vi "reward_behavior_michelle_visjitter_conswin_AllEnticefx.vi"() -> ()   [LabVIEW 2019]
doc: "The myRIO Project template acquires acceleration data from the onboard accelerometer and displays the changes of acceleration values in a waveform chart."
uses:
  <vilib>/myRIO/Common/Instrument Driver Framework/Utilities/typedefs/Generic FPGA Reference.ctl
  <vilib>/myRIO/Common/Instrument Driver Framework/Utilities/typedefs/myRIO v1.0 Reference.ctl
  <vilib>/myRIO/Common/Instrument Driver Framework/Utilities/typedefs/Hardware Version Enum.ctl
  <vilib>/myRIO/Common/Instrument Driver Framework/Utilities/typedefs/myRIO Generic Hardware Reference.ctl
  <vilib>/userdefined/High Color/nirio_resource_hc.ctl
  <vilib>/myRIO/Common/Instrument Driver Framework/Utilities/vis/Is FPGA Ref Available.vi
  <vilib>/myRIO/Common/Instrument Driver Framework/myRIO v1.0/Encoder/typedefs/Encoder Signal Mode.ctl
  <vilib>/myRIO/Common/Instrument Driver Framework/myRIO v1.0/Encoder/typedefs/Encoder Channels Enum.ctl
  <vilib>/myRIO/Instrument Drivers/Onboard IO/Encoder/typedefs/Encoder Reference.ctl
  <vilib>/myRIO/Instrument Drivers/Onboard IO/Encoder/Encoder.lvlib
  <vilib>/myRIO/Instrument Drivers/Onboard IO/Encoder/vis/Read.vi
  <vilib>/myRIO/Common/Instrument Driver Framework/myRIO v1.0/Encoder/typedefs/Encoder Configuration v1.0.ctl
  <vilib>/myRIO/Common/Instrument Driver Framework/myRIO v1.0/Encoder/vis/myRIO v1.1 Open Encoder.vi
  <vilib>/myRIO/Common/Instrument Driver Framework/myRIO v1.0/Encoder/vis/myRIO v1.0 Configure Encoder.vi
  <vilib>/myRIO/Instrument Drivers/Onboard IO/Encoder/vis/myRIO Encoder Open.xnode
  <vilib>/myRIO/Express VI/Onboard IO/Encoder/Encoder Express VI.xnode
  <vilib>/myRIO/Express VI/Onboard IO/DI/DI Express VI.xnode
  <vilib>/myRIO/Instrument Drivers/Onboard IO/DIO/vis/Read.vi
  <vilib>/myRIO/Instrument Drivers/Onboard IO/DIO/DIO.lvlib
  <vilib>/myRIO/Common/Instrument Driver Framework/myRIO v1.0/DIO/typedefs/DIO Channels Enum.ctl
  <vilib>/myRIO/Common/Instrument Driver Framework/myRIO v1.0/DIO/typedefs/DIO Channels List.ctl
  <vilib>/myRIO/Instrument Drivers/Onboard IO/DIO/typedefs/DIO Reference.ctl
  <vilib>/myRIO/Instrument Drivers/Onboard IO/DIO/vis/myRIO DIO Open.xnode
  <vilib>/myRIO/Common/Instrument Driver Framework/myRIO v1.0/DIO/vis/myRIO v1.1 Open DIO.vi
  <vilib>/myRIO/Instrument Drivers/Onboard IO/DIO/vis/Write.vi
  <vilib>/myRIO/Express VI/Onboard IO/DO/DO Express VI.xnode
  <vilib>/Analysis/Matrix/Datatypes/RealMatrix.ctl
  <vilib>/Analysis/Matrix/NI_Matrix.lvlib
panel:
  out "ContrastChoice":dbl
  out "MissCrit":i32
  out "EnticeMatch":i32
  out "CatchVal":i32
  out "Enticements":i32
  in  "Entice":bool
  out "Misses":i32
  out "GoAhead":bool
  out "TimeOutDuration":i32
  out "ActiveTime":dbl
  out "ConsumptionGo":bool=TRUE
  out "Consumption_Period":i32
  out "Watch_Display":bool=TRUE
  in  "Give reward":bool
  out "Timings":dbl[](array[numeric])
  out "ISI":dbl
  out "ISI start time":dbl
  out "Time_out":bool=TRUE
  out "Time since lick":dbl
  out "Time of last lick":dbl
  out "Rewarded trials":dbl[](array[numeric])
  out "Rewards":u16
  out "Active Trial":bool
  out "Array temp2":T1
  out "Stimuli Loaded":bool
  out "Stim_ID":dbl[](array[numeric])
  out "Reward_mat":dbl[](array[numeric])
  out "Reward":bool=TRUE
  out "Frame clock":i32
  out "Licks":u32
  out "Lick":bool
  out "Time":dbl
  out "Stop":bool
  in  "Frames to collect":u32
  out "Overflow?":bool
  out "Counter Value":i32
  out "Velocity":dbl
  out "Velocity Plot":dbl[](graph)
  out "Velocity array":dbl[](array[numeric])
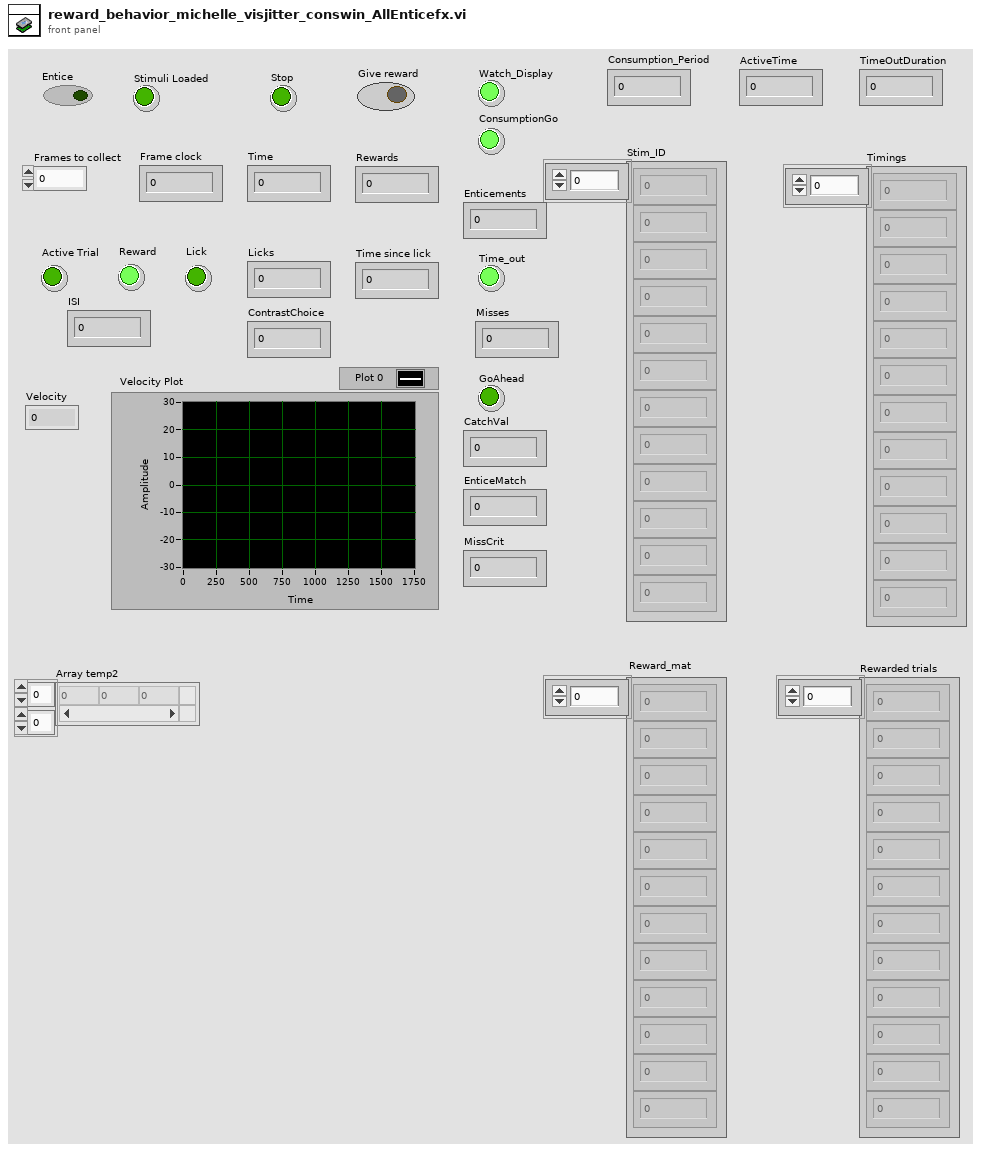
[diagram p1: front panel]
types:
  T1 = typedef "NI_Matrix.lvlib/RealMatrix.ctl" = dbl[][]
  T2 = typedef "Encoder.lvlib/Encoder Reference.ctl" = cluster{"myRIO Reference":T3, "Encoder Channels Enum":T7}
  T3 = typedef "myRIO Generic Hardware Reference.ctl" = cluster{"myRIO Model":T4, "myRIO Hardware Reference":T5}
  T4 = typedef "Hardware Version Enum.ctl" = enum16{"Unknown", "myRIO-1900", "myRIO-1950", "roboRIO", "NI ELVIS RIO CM", "ELVIS III"}
  T5 = typedef "myRIO v1.0 Reference.ctl" = cluster{"Generic FPGA Reference":T6, "Allow multiple opens":bool}
  T6 = typedef "Generic FPGA Reference.ctl" = refnum<k20>
  T7 = typedef "Encoder Channels Enum.ctl" = enum16{"Not Connected", "C/ENC0", "C/ENC1", "A/ENC", "A/ENC0", "A/ENC1", "A/ENC2", "A/ENC3", "A/ENC4", "A/ENC5", "A/ENC6", "A/ENC7", "A/ENC8", "A/ENC9", "B/ENC", "B/ENC0", "B/ENC1", "B/ENC2", "B/ENC3", "B/ENC4", "B/ENC5", "B/ENC6", "B/ENC7", "B/ENC8", "B/ENC9", "DIO/ENC0", "DIO/ENC1", "DIO/ENC2", "DIO/ENC3", "DIO/ENC4"}
  T8 = typedef "Encoder Signal Mode.ctl" = enum16{"Quadrature phase signal", "Step and direction signal"}
  T9 = typedef "nirio_resource_hc.ctl" = tag
  T10 = typedef "DIO.lvlib/DIO Reference.ctl" = cluster{"myRIO Reference":T3, "DIO Channels List":T11}
  T11 = typedef "DIO Channels List.ctl" = T12[]
  T12 = typedef "DIO Channels Enum.ctl" = enum16{"Not Connected", "C/DIO0", "C/DIO1", "C/DIO2", "C/DIO3", "C/DIO4", "C/DIO5", "C/DIO6", "C/DIO7", "A/DIO0", "A/DIO1", "A/DIO2", "A/DIO3", "A/DIO4", "A/DIO5", "A/DIO6", "A/DIO7", "A/DIO8", "A/DIO9", "A/DIO10", "A/DIO11", "A/DIO12", "A/DIO13", "A/DIO14", "A/DIO15", "A/DIO16", "A/DIO17", "A/DIO18", "A/DIO19", "B/DIO0", "B/DIO1", "B/DIO2", "B/DIO3", "B/DIO4", "B/DIO5", "B/DIO6", "B/DIO7", "B/DIO8", "B/DIO9", "B/DIO10", "B/DIO11", "B/DIO12", "B/DIO13", "B/DIO14", "B/DIO15", "B/DIO16", "B/DIO17", "B/DIO18", "B/DIO19", "LED0", "LED1", "LED2", "LED3", "Button0", "DIO/DIO0", "DIO/DIO1", "DIO/DIO2", "DIO/DIO3", "DIO/DIO4", "DIO/DIO5", "DIO/DIO6", "DIO/DIO7", "DIO/DIO8", "DIO/DIO9", "SPI/CS0", "SPI/CS1", "SPI/CS2", "SPI/CS3", "LED RADIO (Green)", "LED RADIO (Red)", "LED COMM (Green)", "LED COMM (Red)", "LED MODE (Green)", "LED MODE (Red)"}
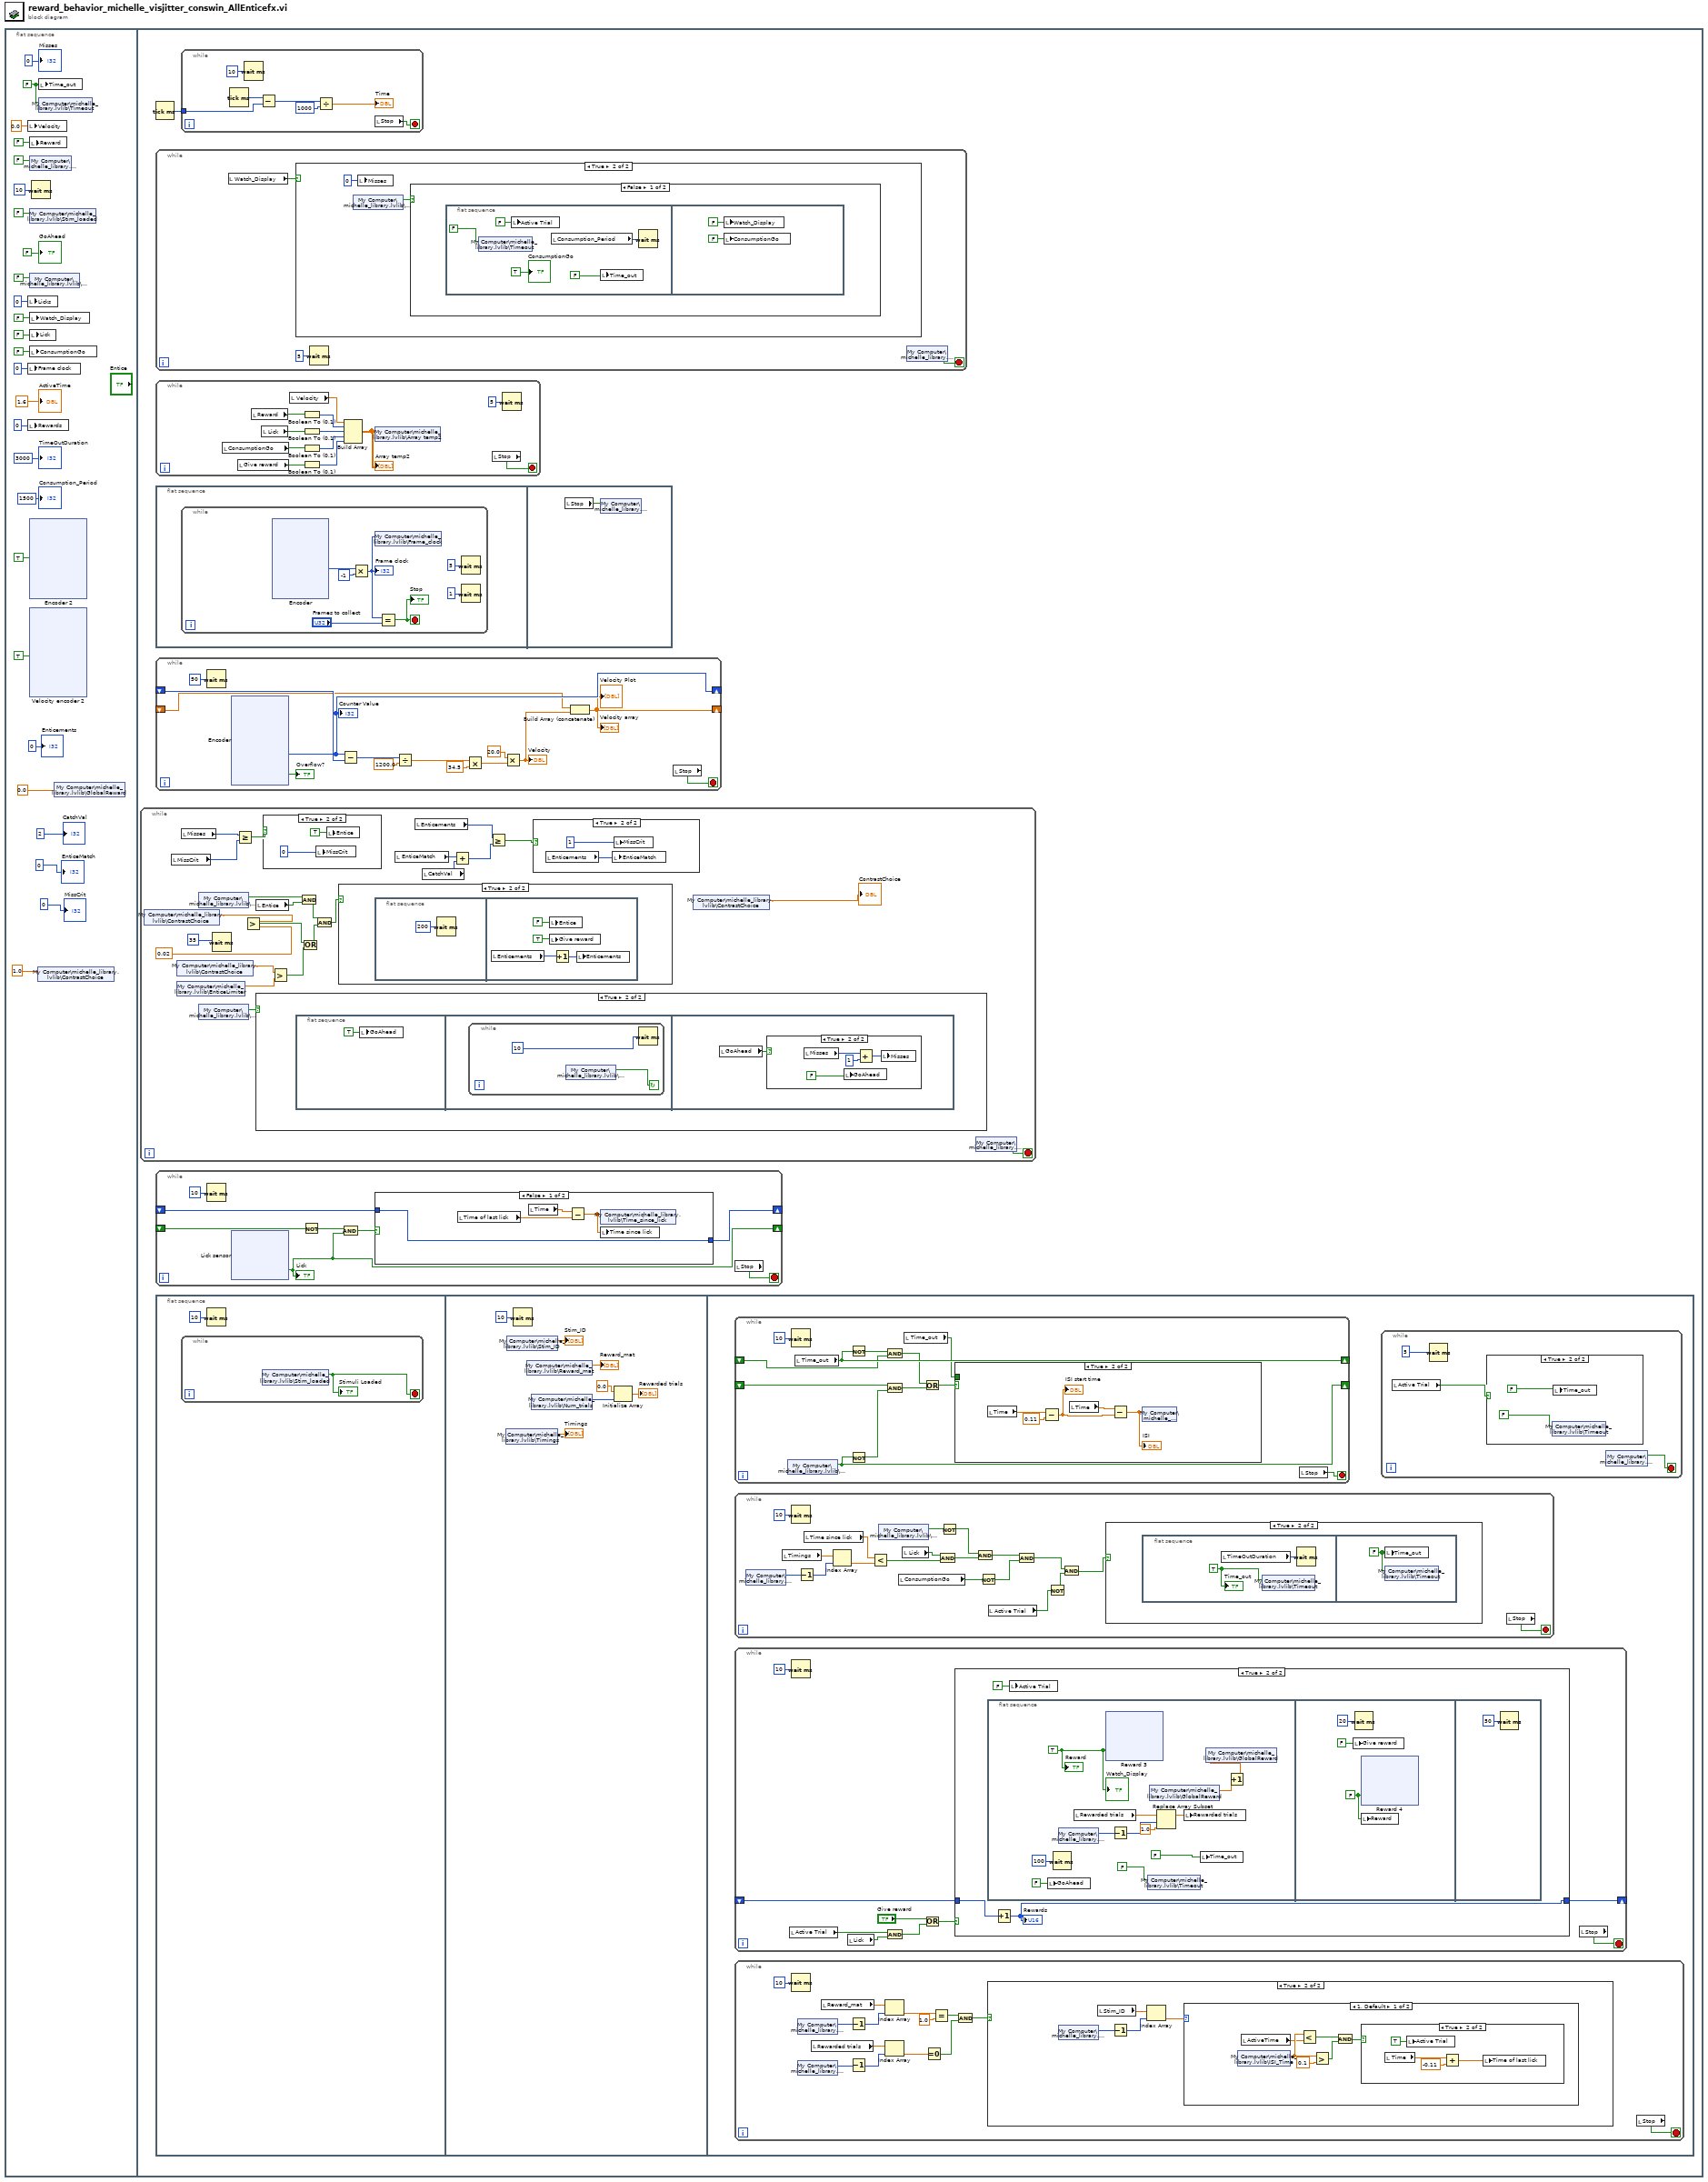
[diagram p0: block diagram]
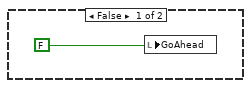
[diagram p5: hidden frame]
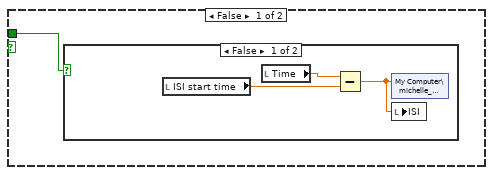
[diagram p11: hidden frame]
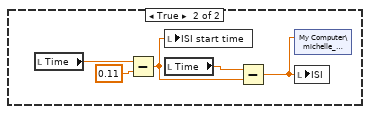
[diagram p12: hidden frame]
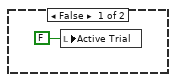
[diagram p13: hidden frame]
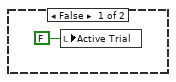
[diagram p14: hidden frame]
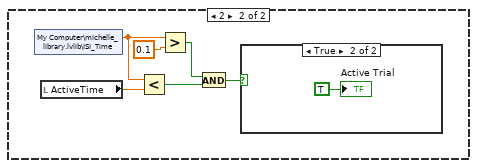
[diagram p15: hidden frame]
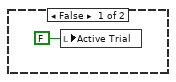
[diagram p16: hidden frame]
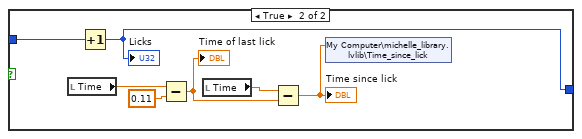
[diagram p18: hidden frame]
diagram:
  n1 = flat-sequence {
    frame #0 {
      w14 = FALSE ("Time_out")
      n2 = local write "Velocity"(0.0 ("Velocity")) -> ()
      n3 = local write "Licks"(u32 0 ("Licks")) -> ()
      n4 = local write "Frame clock"(u32 0 ("Frames")) -> ()
      n5 = local write "Rewards"(u16 0 ("Rewards")) -> ()
      n6 = local write "Reward"(FALSE ("Give reward")) -> ()
      n7 = shared-variable "My Computer\\michelle_library.lvlib\\Stop"(FALSE ("Stop")) -> ()  [unwired: 1 in, 1 out]
      n8 = shared-variable "My Computer\\michelle_library.lvlib\\Stim_loaded"(FALSE ("Stim_loaded")) -> ()  [unwired: 1 in, 1 out]
      n9 = shared-variable "My Computer\\michelle_library.lvlib\\Display"(FALSE ("Display")) -> ()  [unwired: 1 in, 1 out]
      n10 = local write "Watch_Display"(FALSE ("Watch_Display")) -> ()
      n11 = local write "Lick"(FALSE ("Lick")) -> ()
      n12 = local write "ConsumptionGo"(FALSE ("ConsumptionGo")) -> ()
      n13 = xnode "Encoder 2"("Reset Counter"=TRUE) -> ()  [unwired: 1 in, 4 out]
      n14 = xnode "Velocity encoder 2"("Reset Counter"=TRUE) -> ()  [unwired: 1 in, 4 out]
      n15 = Wait (ms)(milliseconds to wait=u32 10) -> ()  [unwired: 1 out]
      n16 = shared-variable "My Computer\\michelle_library.lvlib\\ContrastChoice"(1.0) -> ()  [unwired: 1 in, 1 out]
      n17 = local write "Time_out"(w14) -> ()
      n18 = shared-variable "My Computer\\michelle_library.lvlib\\Timeout"(w14) -> ()  [unwired: 1 in, 1 out]
      n19 = shared-variable "My Computer\\michelle_library.lvlib\\GlobalReward"(0.0) -> ()  [unwired: 1 in, 1 out]
      "Consumption_Period" <- 1500
      "ActiveTime" <- 1.6
      "TimeOutDuration" <- 3000
      "GoAhead" <- FALSE
      "Misses" <- 0
      "Enticements" <- 0
      "CatchVal" <- 2
      "EnticeMatch" <- 0
      "MissCrit" <- 0
    }
    frame #1 {
      n20 = while {
        stop <- w142 stop-if-true
        n21 = shared-variable "My Computer\\michelle_library.lvlib\\ContrastChoice"() -> (w129:dbl)  [unwired: 1 in, 1 out]
        n22 = local read "MissCrit"() -> (w130:i32)
        n23 = shared-variable "My Computer\\michelle_library.lvlib\\ContrastChoice"() -> (w121:dbl)  [unwired: 1 in, 1 out]
        n24 = shared-variable "My Computer\\michelle_library.lvlib\\EnticeLimiter"() -> (w120:dbl)  [unwired: 1 in, 1 out]
        n25 = local read "Misses"() -> (w136:i32)
        n26 = shared-variable "My Computer\\michelle_library.lvlib\\Display"() -> (w140:bool)  [unwired: 1 in, 1 out]
        n27 = shared-variable "My Computer\\michelle_library.lvlib\\Display"() -> (w141:bool)  [unwired: 1 in, 1 out]
        n28 = Wait (ms)(milliseconds to wait=35) -> ()  [unwired: 1 out]
        n29 = Greater Or Equal?(x=w136, y=w130) -> (x >= y?=w137:bool)
        n30 = Greater?(x=w129, y=0.02) -> (0:w123:bool)
        n31 = local read "Entice"() -> (w139:bool)
        n32 = case shown="True" w141 {
          frame False {
            n33 = local write "GoAhead"(FALSE) -> ()
          }
          frame True {
            n34 = flat-sequence {
              frame #0 {
                n35 = local write "GoAhead"(TRUE) -> ()
              }
              frame #1 {
                n36 = while {
                  stop <- w155 continue-if-true
                  n37 = shared-variable "My Computer\\michelle_library.lvlib\\Display"() -> (w155:bool)  [unwired: 1 in, 1 out]
                  n38 = Wait (ms)(milliseconds to wait=10) -> ()  [unwired: 1 out]
                }
              }
              frame #2 {
                n39 = local read "GoAhead"() -> (w156:bool)
                n40 = case shown="True" w156 {
                  frame False {
                  }
                  frame True {
                    n41 = local read "Misses"() -> (w160:i32)
                    n42 = local write "GoAhead"(FALSE) -> ()
                    n43 = Add(x=w160, y=1) -> (x+y=w158:i32)
                    n44 = local write "Misses"(w158) -> ()
                  }
                }
              }
            }
          }
        }
        n45 = case shown="True" w137 {
          frame False {
          }
          frame True {
            n46 = local write "MissCrit"(0) -> ()
            n47 = local write "Entice"(TRUE) -> ()
          }
        }
        n48 = Greater?(x=w121, y=w120) -> (0:w122:bool)
        n49 = And(x=w140, y=w139) -> (x .and. y?=w127:bool)
        n50 = Or(x=w123, y=w122) -> (x .or. y?=w124:bool)
        n51 = And(x=w127, y=w124) -> (x .and. y?=w126:bool)
        n52 = case shown="True" w126 {
          frame False {
          }
          frame True {
            n53 = flat-sequence {
              frame #0 {
                n54 = Wait (ms)(milliseconds to wait=200) -> ()  [unwired: 1 out]
              }
              frame #1 {
                n55 = local read "Enticements"() -> (w147:i32)
                n56 = local write "Entice"(FALSE) -> ()
                n57 = local write "Give reward"(TRUE) -> ()
                n58 = Increment(x=w147) -> (x+1=w146:i32)
                n59 = local write "Enticements"(w146) -> ()
              }
            }
          }
        }
        n60 = local read "EnticeMatch"() -> (w133:i32)
        n61 = local read "Enticements"() -> (w135:i32)
        n62 = local read "CatchVal"() -> (w134:i32)
        n63 = Add(x=w133, y=w134) -> (x+y=w132:i32)
        n64 = Greater Or Equal?(x=w135, y=w132) -> (x >= y?=w131:bool)
        n65 = case shown="True" w131 {
          frame False {
          }
          frame True {
            n66 = local read "Enticements"() -> (w143:i32)
            n67 = local write "EnticeMatch"(w143) -> ()
            n68 = local write "MissCrit"(1) -> ()
          }
        }
        n69 = shared-variable "My Computer\\michelle_library.lvlib\\ContrastChoice"() -> (→"ContrastChoice":dbl)  [unwired: 1 in, 1 out]
        n70 = shared-variable "My Computer\\michelle_library.lvlib\\Stop"() -> (w142:bool)  [unwired: 1 in, 1 out]
      }
      n71 = Tick Count (ms)() -> (millisecond timer value=w119:u32)
      n72 = while {
        stop <- w163 stop-if-true
        n73 = local read "Watch_Display"() -> (w162:bool)
        n74 = case shown="True" w162 {
          frame False {
          }
          frame True {
            n75 = shared-variable "My Computer\\michelle_library.lvlib\\Display"() -> (w165:bool)  [unwired: 1 in, 1 out]
            n76 = local write "Misses"(0) -> ()
            n77 = case shown="False" w165 {
              frame False {
                n78 = flat-sequence {
                  frame #0 {
                    n79 = shared-variable "My Computer\\michelle_library.lvlib\\Timeout"(FALSE) -> ()  [unwired: 1 in, 1 out]
                    n80 = local write "Active Trial"(FALSE) -> ()
                    n81 = local read "Consumption_Period"() -> (w170:i32)
                    n82 = local write "Time_out"(FALSE) -> ()
                    n83 = Wait (ms)(milliseconds to wait=w170) -> ()  [unwired: 1 out]
                    "ConsumptionGo" <- TRUE
                  }
                  frame #1 {
                    n84 = local write "Watch_Display"(FALSE ("Watch_Display")) -> ()
                    n85 = local write "ConsumptionGo"(FALSE ("ConsumptionGo")) -> ()
                  }
                }
              }
              frame True {
              }
            }
          }
        }
        n86 = Wait (ms)(milliseconds to wait=u32 5) -> ()  [unwired: 1 out]
        n87 = shared-variable "My Computer\\michelle_library.lvlib\\Stop"() -> (w163:bool)  [unwired: 1 in, 1 out]
      }
      n88 = while {
        stop <- w178 stop-if-true
        n89 = local read "ConsumptionGo"() -> (w176:bool)
        n90 = local read "Give reward"() -> (w175:bool)
        n91 = local read "Reward"() -> (w183:bool)
        n92 = local read "Lick"() -> (w184:bool)
        n93 = local read "Velocity"() -> (w182:dbl)
        n94 = Boolean To (0,1)(Boolean=w183) -> (0, 1=w181:i16)
        n95 = Boolean To (0,1)(Boolean=w184) -> (0, 1=w180:i16)
        n96 = Boolean To (0,1)(Boolean=w176) -> (0, 1=w174:i16)
        n97 = Boolean To (0,1)(Boolean=w175) -> (0, 1=w173:i16)
        n98 = Build Array(w182, w181, w180, w174, w173) -> (w177:T1)
        "Array temp2" <- w177
        n99 = shared-variable "My Computer\\michelle_library.lvlib\\Array temp2"(w177) -> ()  [unwired: 1 in, 1 out]
        n100 = local read "Stop"() -> (w178:bool)
        n101 = Wait (ms)(milliseconds to wait=u32 5) -> ()  [unwired: 1 out]
      }
      n102 = flat-sequence {
        frame #0 {
          n103 = while {
            stop <- w385 stop-if-true
            n104 = xnode "Encoder"() -> ("Counter Value"=w389:i32)  [unwired: 2 in, 3 out]
            n105 = Multiply(x=w389, y=-1) -> (x*y=w384:i32)
            "Frame clock" <- w384
            n106 = shared-variable "My Computer\\michelle_library.lvlib\\Frame_clock"(w384) -> ()  [unwired: 1 in, 1 out]
            n107 = Equal?(x=w384, y="Frames to collect") -> (x = y?=w385:bool)
            "Stop" <- w385
            n108 = Wait (ms)(milliseconds to wait=u32 5) -> ()  [unwired: 1 out]
            n109 = Wait (ms)(milliseconds to wait=u32 1) -> ()  [unwired: 1 out]
          }
        }
        frame #1 {
          n110 = local read "Stop"() -> (w437:bool)
          n111 = shared-variable "My Computer\\michelle_library.lvlib\\Stop"(w437) -> ()  [unwired: 1 in, 1 out]
        }
      }
      n112 = while {
        shift-right: [w502] -> _
        shift-left: _ -> [w503]
        shift-right: [w494] -> _
        shift-left: _ -> [w493]
        stop <- w492 stop-if-true
        n113 = Wait (ms)(milliseconds to wait=u32 50) -> ()  [unwired: 1 out]
        n114 = xnode "Encoder"() -> ("Counter Value"=w502:i32, "Overflow?"=→"Overflow?":bool)  [unwired: 2 in, 2 out]
        "Counter Value" <- w502
        n115 = Subtract(x=w502, y=w503) -> (x-y=w495:i32)
        n116 = Divide(x=w495, y=1200.0 ("600")) -> (x/y=w500:dbl)
        n117 = Multiply(x=w500, y=34.5) -> (x*y=w498:dbl)
        n118 = Multiply(x=20.0, y=w498) -> (x*y=w496:dbl)
        "Velocity" <- w496
        n119 = Build Array (concatenate)(w493, w496) -> (w494:dbl[])
        "Velocity Plot" <- w494
        "Velocity array" <- w494
        n120 = local read "Stop"() -> (w492:bool)
      }
      n121 = while {
        shift-right: [w444] -> _
        shift-left: _ -> [w443]
        shift-right: [w438] -> _
        shift-left: _ -> [w441]
        stop <- w442 stop-if-true
        n122 = Wait (ms)(milliseconds to wait=u32 10) -> ()  [unwired: 1 out]
        n123 = xnode "Lick sensor"() -> ("C/DIO1 (DIO1)"=w438:bool)  [unwired: 1 in, 1 out]
        "Lick" <- w438
        n124 = Not(x=w441) -> (.not. x?=w440:bool)
        n125 = And(x=w440, y=w438) -> (x .and. y?=w439:bool)
        n126 = case shown="False" w439 {
          tunnel: [w449 w456] -> w444
          tunnel: w443 -> [w449 w455]
          frame False {
            n127 = local read "Time of last lick"() -> (w447:dbl)
            n128 = local read "Time"() -> (w448:dbl)
            n129 = Subtract(x=w448, y=w447) -> (x-y=w446:dbl)
            n130 = shared-variable "My Computer\\michelle_library.lvlib\\Time_since_lick"(w446) -> ()  [unwired: 1 in, 1 out]
            n131 = local write "Time since lick"(w446) -> ()
          }
          frame True {
            n132 = local read "Time"() -> (w452:dbl)
            n133 = Increment(x=w455) -> (x+1=w456:u32)
            "Licks" <- w456
            n134 = Subtract(x=w452, y=0.11) -> (x-y=w450:dbl)
            "Time of last lick" <- w450
            n135 = local read "Time"() -> (w454:dbl)
            n136 = Subtract(x=w454, y=w450) -> (x-y=w453:dbl)
            "Time since lick" <- w453
            n137 = shared-variable "My Computer\\michelle_library.lvlib\\Time_since_lick"(w453) -> ()  [unwired: 1 in, 1 out]
          }
        }
        n138 = local read "Stop"() -> (w442:bool)
      }
      n139 = flat-sequence {
        frame #0 {
          n140 = while {
            stop <- w186 stop-if-true
            n141 = shared-variable "My Computer\\michelle_library.lvlib\\Stim_loaded"() -> (w186:bool)  [unwired: 1 in, 1 out]
            "Stimuli Loaded" <- w186
          }
          n142 = Wait (ms)(milliseconds to wait=u32 10) -> ()  [unwired: 1 out]
        }
        frame #1 {
          n143 = shared-variable "My Computer\\michelle_library.lvlib\\Timings"() -> (→"Timings":dbl[])  [unwired: 1 in, 1 out]
          n144 = shared-variable "My Computer\\michelle_library.lvlib\\Stim_ID"() -> (→"Stim_ID":dbl[])  [unwired: 1 in, 1 out]
          n145 = Wait (ms)(milliseconds to wait=u32 10) -> ()  [unwired: 1 out]
          n146 = shared-variable "My Computer\\michelle_library.lvlib\\Reward_mat"() -> (→"Reward_mat":dbl[])  [unwired: 1 in, 1 out]
          n147 = shared-variable "My Computer\\michelle_library.lvlib\\Num_trials"() -> (w190:u32)  [unwired: 1 in, 1 out]
          n148 = Initialize Array(0.0 ("element"), w190) -> (→"Rewarded trials":dbl[])
        }
        frame #2 {
          n149 = while {
            shift-right: [w231] -> _
            shift-left: _ -> [w229]
            shift-right: [w227] -> _
            shift-left: _ -> [w226]
            stop <- w232 stop-if-true
            n150 = shared-variable "My Computer\\michelle_library.lvlib\\Display"() -> (w227:bool)  [unwired: 1 in, 1 out]
            n151 = Wait (ms)(milliseconds to wait=u32 10) -> ()  [unwired: 1 out]
            n152 = local read "Time_out"() -> (w231:bool)
            n153 = Not(x=w231) -> (.not. x?=w230:bool)
            n154 = Not(x=w227) -> (.not. x?=w225:bool)
            n155 = And(x=w230, y=w229) -> (x .and. y?=w224:bool)
            n156 = And(x=w226, y=w225) -> (x .and. y?=w223:bool)
            n157 = local read "Time_out"() -> (w228:bool)
            n158 = Or(x=w224, y=w223) -> (x .or. y?=w222:bool)
            n159 = case shown="True" w222 {
              tunnel: w228 -> [w233 _]
              frame False {
                n160 = case shown="False" w233 {
                  frame False {
                    n161 = local read "ISI start time"() -> (w236:dbl)
                    n162 = local read "Time"() -> (w235:dbl)
                    n163 = Subtract(x=w235, y=w236) -> (x-y=w234:dbl)
                    n164 = shared-variable "My Computer\\michelle_library.lvlib\\ISI"(w234) -> ()  [unwired: 1 in, 1 out]
                    n165 = local write "ISI"(w234) -> ()
                  }
                  frame True {
                    n166 = local read "Time"() -> (w241:dbl)
                    n167 = Subtract(x=w241, y=0.11) -> (x-y=w238:dbl)
                    n168 = local write "ISI start time"(w238) -> ()
                    n169 = local read "Time"() -> (w239:dbl)
                    n170 = Subtract(x=w239, y=w238) -> (x-y=w237:dbl)
                    n171 = shared-variable "My Computer\\michelle_library.lvlib\\ISI"(w237) -> ()  [unwired: 1 in, 1 out]
                    n172 = local write "ISI"(w237) -> ()
                  }
                }
              }
              frame True {
                n173 = local read "Time"() -> (w246:dbl)
                n174 = Subtract(x=w246, y=0.11) -> (x-y=w243:dbl)
                "ISI start time" <- w243
                n175 = local read "Time"() -> (w244:dbl)
                n176 = Subtract(x=w244, y=w243) -> (x-y=w242:dbl)
                "ISI" <- w242
                n177 = shared-variable "My Computer\\michelle_library.lvlib\\ISI"(w242) -> ()  [unwired: 1 in, 1 out]
              }
            }
            n178 = local read "Stop"() -> (w232:bool)
          }
          n179 = while {
            stop <- w217 stop-if-true
            n180 = shared-variable "My Computer\\michelle_library.lvlib\\Trial"() -> (w207:u32)  [unwired: 1 in, 1 out]
            n181 = local read "Timings"() -> (w209:dbl[])
            n182 = Wait (ms)(milliseconds to wait=u32 10) -> ()  [unwired: 1 out]
            n183 = Decrement(x=w207) -> (x-1=w206:u32)
            n184 = local read "Time since lick"() -> (w216:dbl)
            n185 = Index Array(array=w209, index=w206) -> (element=w208:dbl)
            n186 = Less?(x=w216, y=w208) -> (x < y?=w215:bool)
            n187 = shared-variable "My Computer\\michelle_library.lvlib\\Display"() -> (w212:bool)  [unwired: 1 in, 1 out]
            n188 = local read "ConsumptionGo"() -> (w204:bool)
            n189 = local read "Lick"() -> (w214:bool)
            n190 = And(x=w214, y=w215) -> (x .and. y?=w210:bool)
            n191 = Not(x=w212) -> (.not. x?=w211:bool)
            n192 = And(x=w211, y=w210) -> (x .and. y?=w203:bool)
            n193 = Not(x=w204) -> (.not. x?=w205:bool)
            n194 = local read "Active Trial"() -> (w199:bool)
            n195 = And(x=w203, y=w205) -> (x .and. y?=w201:bool)
            n196 = Not(x=w199) -> (.not. x?=w202:bool)
            n197 = And(x=w201, y=w202) -> (x .and. y?=w200:bool)
            n198 = case shown="True" w200 {
              frame False {
              }
              frame True {
                n199 = flat-sequence {
                  frame #0 {
                    w219 = TRUE
                    n200 = local read "TimeOutDuration"() -> (w218:i32)
                    n201 = shared-variable "My Computer\\michelle_library.lvlib\\Timeout"(w219) -> ()  [unwired: 1 in, 1 out]
                    n202 = Wait (ms)(milliseconds to wait=w218) -> ()  [unwired: 1 out]
                    "Time_out" <- w219
                  }
                  frame #1 {
                    w220 = FALSE ("Timeout")
                    n203 = local write "Time_out"(w220) -> ()
                    n204 = shared-variable "My Computer\\michelle_library.lvlib\\Timeout"(w220) -> ()  [unwired: 1 in, 1 out]
                  }
                }
              }
            }
            n205 = local read "Stop"() -> (w217:bool)
          }
          n206 = while {
            shift-right: [w291] -> _
            shift-left: _ -> [w290]
            stop <- w293 stop-if-true
            n207 = local read "Active Trial"() -> (w288:bool)
            n208 = Wait (ms)(milliseconds to wait=u32 10) -> ()  [unwired: 1 out]
            n209 = local read "Lick"() -> (w289:bool)
            n210 = And(x=w288, y=w289) -> (x .and. y?=w287:bool)
            n211 = Or(x="Give reward", y=w287) -> (x .or. y?=w286:bool)
            n212 = case shown="True" w286 {
              tunnel: [w294 w297] -> w291
              tunnel: w290 -> [w294 w296]
              frame False {
              }
              frame True {
                n213 = flat-sequence {
                  frame #0 {
                    w308 = TRUE ("C/DIO0 (DIO0)")
                    n214 = local write "GoAhead"(FALSE) -> ()
                    n215 = Wait (ms)(milliseconds to wait=u32 100) -> ()  [unwired: 1 out]
                    n216 = shared-variable "My Computer\\michelle_library.lvlib\\Trial"() -> (w307:u32)  [unwired: 1 in, 1 out]
                    n217 = local read "Rewarded trials"() -> (w305:dbl[])
                    n218 = xnode "Reward 3"("C/DIO0 (DIO0)"=w308) -> ()  [unwired: 1 in, 1 out]
                    n219 = Decrement(x=w307) -> (x-1=w306:u32)
                    n220 = shared-variable "My Computer\\michelle_library.lvlib\\Timeout"(FALSE) -> ()  [unwired: 1 in, 1 out]
                    n221 = shared-variable "My Computer\\michelle_library.lvlib\\GlobalReward"() -> (w299:dbl)  [unwired: 1 in, 1 out]
                    n222 = Replace Array Subset(array=w305, new element=1.0 ("new element/subarray"), index=w306) -> (w303:dbl[])
                    n223 = local write "Rewarded trials"(w303) -> ()
                    n224 = local write "Time_out"(FALSE) -> ()
                    n225 = Increment(x=w299) -> (x+1=w298:dbl)
                    n226 = shared-variable "My Computer\\michelle_library.lvlib\\GlobalReward"(w298) -> ()  [unwired: 1 in, 1 out]
                    "Reward" <- w308
                    "Watch_Display" <- w308
                  }
                  frame #1 {
                    w347 = FALSE ("C/DIO0 (DIO0)")
                    n227 = local write "Give reward"(FALSE ("Give reward")) -> ()
                    n228 = Wait (ms)(milliseconds to wait=u32 20) -> ()  [unwired: 1 out]
                    n229 = xnode "Reward 4"("C/DIO0 (DIO0)"=w347) -> ()  [unwired: 1 in, 1 out]
                    n230 = local write "Reward"(w347) -> ()
                  }
                  frame #2 {
                    n231 = Wait (ms)(milliseconds to wait=u32 50) -> ()  [unwired: 1 out]
                  }
                }
                n232 = Increment(x=w296) -> (x+1=w297:u16)
                "Rewards" <- w297
                n233 = local write "Active Trial"(FALSE ("Active Trial")) -> ()
              }
            }
            n234 = local read "Stop"() -> (w293:bool)
          }
          n235 = while {
            stop <- w260 stop-if-true
            n236 = Wait (ms)(milliseconds to wait=u32 10) -> ()  [unwired: 1 out]
            n237 = shared-variable "My Computer\\michelle_library.lvlib\\Trial"() -> (w256:u32)  [unwired: 1 in, 1 out]
            n238 = shared-variable "My Computer\\michelle_library.lvlib\\Trial"() -> (w252:u32)  [unwired: 1 in, 1 out]
            n239 = local read "Rewarded trials"() -> (w253:dbl[])
            n240 = local read "Reward_mat"() -> (w255:dbl[])
            n241 = Decrement(x=w256) -> (x-1=w257:u32)
            n242 = Decrement(x=w252) -> (x-1=w251:u32)
            n243 = Index Array(array=w255, index=w257) -> (element=w258:dbl)
            n244 = Index Array(array=w253, index=w251) -> (element=w250:dbl)
            n245 = Equal To 0?(x=w250) -> (x = 0?=w249:bool)
            n246 = Equal?(x=w258, y=1.0) -> (x = y?=w248:bool)
            n247 = And(x=w248, y=w249) -> (x .and. y?=w247:bool)
            n248 = case shown="True" w247 {
              frame False {
                n249 = local write "Active Trial"(FALSE ("Active_trial")) -> ()
              }
              frame True {
                n250 = shared-variable "My Computer\\michelle_library.lvlib\\Trial"() -> (w263:u32)  [unwired: 1 in, 1 out]
                n251 = local read "Stim_ID"() -> (w265:dbl[])
                n252 = Decrement(x=w263) -> (x-1=w264:u32)
                n253 = Index Array(array=w265, index=w264) -> (element=w262:dbl)
                n254 = case shown="1, Default" w262 {
                  frame 1, Default {
                    n255 = shared-variable "My Computer\\michelle_library.lvlib\\ISI_Time"() -> (w271:dbl)  [unwired: 1 in, 1 out]
                    n256 = local read "ActiveTime"() -> (w266:dbl)
                    n257 = Less?(x=w271, y=w266) -> (x < y?=w269:bool)
                    n258 = Greater?(x=w271, y=0.1) -> (0:w268:bool)
                    n259 = And(x=w269, y=w268) -> (x .and. y?=w267:bool)
                    n260 = case shown="True" w267 {
                      frame False {
                        n261 = local write "Active Trial"(FALSE ("Active Trial")) -> ()
                      }
                      frame True {
                        n262 = local read "Time"() -> (w275:dbl)
                        n263 = local write "Active Trial"(TRUE ("Active Trial")) -> ()
                        n264 = Add(x=w275, y=-0.11) -> (x+y=w273:dbl)
                        n265 = local write "Time of last lick"(w273) -> ()
                      }
                    }
                  }
                  frame 2 {
                    n266 = shared-variable "My Computer\\michelle_library.lvlib\\ISI_Time"() -> (w281:dbl)  [unwired: 1 in, 1 out]
                    n267 = local read "ActiveTime"() -> (w277:dbl)
                    n268 = Less?(x=w281, y=w277) -> (x < y?=w279:bool)
                    n269 = Greater?(x=w281, y=0.1) -> (0:w280:bool)
                    n270 = And(x=w280, y=w279) -> (x .and. y?=w278:bool)
                    n271 = case shown="True" w278 {
                      frame False {
                        n272 = local write "Active Trial"(FALSE ("Active Trial")) -> ()
                      }
                      frame True {
                        "Active Trial" <- TRUE ("Active Trial")
                      }
                    }
                  }
                }
              }
            }
            n273 = local read "Stop"() -> (w260:bool)
          }
          n274 = while {
            stop <- w196 stop-if-true
            n275 = local read "Active Trial"() -> (w195:bool)
            n276 = Wait (ms)(milliseconds to wait=5) -> ()  [unwired: 1 out]
            n277 = case shown="True" w195 {
              frame False {
              }
              frame True {
                n278 = shared-variable "My Computer\\michelle_library.lvlib\\Timeout"(FALSE) -> ()  [unwired: 1 in, 1 out]
                n279 = local write "Time_out"(FALSE) -> ()
              }
            }
            n280 = shared-variable "My Computer\\michelle_library.lvlib\\Stop"() -> (w196:bool)  [unwired: 1 in, 1 out]
          }
        }
      }
      n281 = while {
        tunnel: w119 -> [w557]
        stop <- w555 stop-if-true
        n282 = Tick Count (ms)() -> (millisecond timer value=w558:u32)
        n283 = Wait (ms)(milliseconds to wait=u32 10) -> ()  [unwired: 1 out]
        n284 = Subtract(x=w558, y=w557) -> (x-y=w554:u32)
        n285 = Divide(x=w554, y=u32 1000) -> (x/y=→"Time":dbl)
        n286 = local read "Stop"() -> (w555:bool)
      }
    }
  }
